vi "Create Sample Pressure Curves.vi"() -> ()   [LabVIEW 2020]
panel:
  in  "Length":i32=115
  out "Waveform Graph":dbl[][](graph)
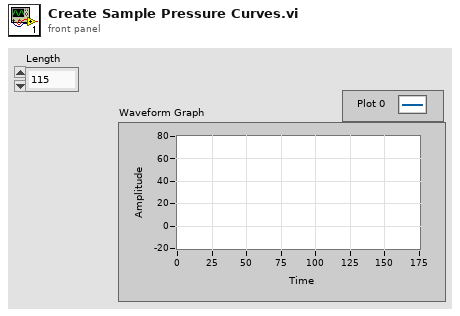
[diagram p1: front panel]
types:
  T1 = enum16{"open", "replace", "create", "open or create", "replace or create", "replace or create with confirmation"}
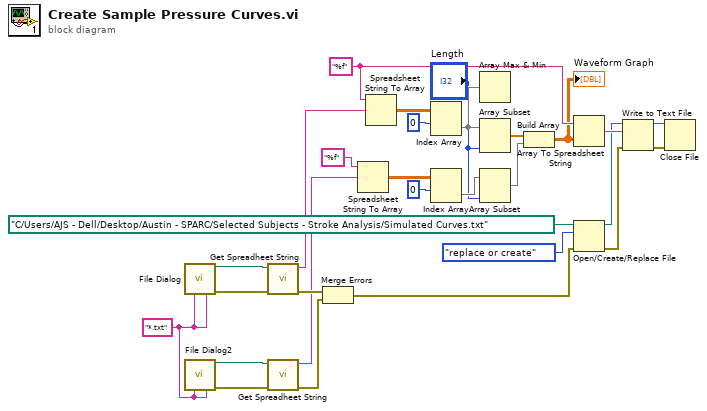
[diagram p0: block diagram]
diagram:
  w14 = "*.txt" ("pattern label")
  w25 = "%f" ("format string")
  n1 = call "File Dialog"("pattern (all files)"=w14, "pattern label"=w14) -> ("selected path"=w29:path, "error out"=w11:errorcluster)  [unwired: 10 in, 2 out]
  n2 = call "File Dialog2"("pattern (all files)"=w14, "pattern label"=w14) -> ("selected path"=w2:path, "error out"=w13:errorcluster)  [unwired: 10 in, 2 out]
  n3 = call "Get Spreadheet String.vi"("error in (no error)"=w11, "File Path"=w29) -> ("error out"=w12:errorcluster, "Spreadsheet String"=w28:string)  [unwired: 8 in]
  n4 = call "Get Spreadheet String.vi"("error in (no error)"=w13, "File Path"=w2) -> ("error out"=w10:errorcluster, "Spreadsheet String"=w3:string)  [unwired: 8 in]
  n5 = Merge Errors(w12, w10) -> (w1:errorcluster)
  n6 = Spreadsheet String To Array(format string="%f", spreadsheet string=w3) -> (array=w9:dbl[][])  [unwired: 2 in]
  n7 = Spreadsheet String To Array(format string=w25, spreadsheet string=w28) -> (array=w27:dbl[][])  [unwired: 2 in]
  n8 = Index Array(array=w27, index (row)=0) -> (element=w16:dbl[])  [unwired: 1 in]
  n9 = Index Array(array=w9, index (row)=0) -> (element=w6:dbl[])  [unwired: 1 in]
  n10 = Array Max & Min(array=w16) -> ()  [unwired: 4 out]
  n11 = Array Subset(array=w16, length="Length") -> (w15:dbl[])  [unwired: 1 in]
  n12 = Array Subset(array=w6, length="Length") -> (w4:dbl[])  [unwired: 1 in]
  n13 = Build Array(w15, w4) -> (w24:dbl[][])
  "Waveform Graph" <- w24
  n14 = Array To Spreadsheet String(array=w24, 3:w25) -> (spreadsheet string=w22:string)  [unwired: 1 in]
  n15 = Open/Create/Replace File(file path (use dialog)=path "C:/Users/AJS - Dell/Desktop/Austin - SPARC/Selected Subjects - Stroke Analysis/Simulated Curves.txt", error in=w1, operation (0:open)=T1."replace or create") -> (refnum out=w21:refnum<file>, error out=w23:errorcluster)  [unwired: 3 in, 1 out]
  n16 = Write to Text File(file (use dialog)=w21, text=w22, error in=w23) -> (refnum out=w19:refnum<file>, error out=w20:errorcluster)  [unwired: 1 in, 1 out]
  n17 = Close File(refnum=w19, error in=w20) -> ()  [unwired: 2 out]
